vi "digit_to_color.vi"() -> ()   [LabVIEW 2018]
uses:
  Digit.ctl
panel:
  out "Color Box":u32(colorbox)=14778368
  in  "Digit":T1
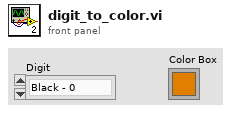
[diagram p1: front panel]
types:
  T1 = typedef "Digit.ctl" = enum16{"Black - 0", "Brown - 1", "Red - 2", "Orange - 3", "Yellow - 4", "Green - 5", "Blue - 6", "Violet - 7", "Grey - 8", "White - 9"}
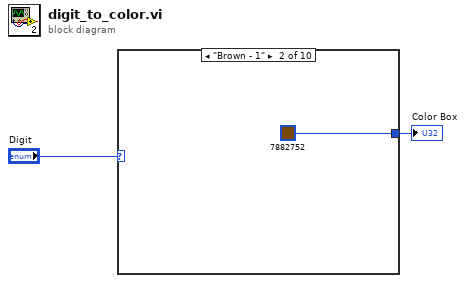
[diagram p0: block diagram]
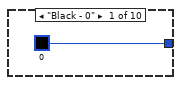
[diagram p2: hidden frame]
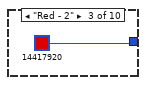
[diagram p3: hidden frame]
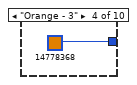
[diagram p4: hidden frame]
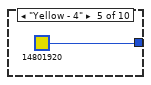
[diagram p5: hidden frame]
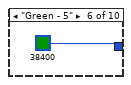
[diagram p6: hidden frame]
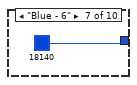
[diagram p7: hidden frame]
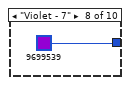
[diagram p8: hidden frame]
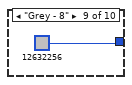
[diagram p9: hidden frame]
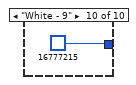
[diagram p10: hidden frame]
diagram:
  n1 = case shown="\"Brown - 1\"" "Digit" {
    tunnel: [u32 0 u32 7882752 u32 14417920 u32 14778368 u32 14801920 u32 38400 u32 18140 u32 9699539 u32 12632256 u32 16777215] -> w1
    frame "Black - 0" {
    }
    frame "Brown - 1" {
    }
    frame "Red - 2" {
    }
    frame "Orange - 3" {
    }
    frame "Yellow - 4" {
    }
    frame "Green - 5" {
    }
    frame "Blue - 6" {
    }
    frame "Violet - 7" {
    }
    frame "Grey - 8" {
    }
    frame "White - 9" {
    }
  }
  "Color Box" <- w1
